vi "PDU Test Program.vi"() -> ()   [LabVIEW 2022 SP3, in "Power Distribution.lvclass"]
uses:
  Power Distribution.lvclass
  Orion PDU/Orion PDU.lvclass
  Power Distribution.lvclass/Power Distribution.ctl
panel:
  in  "Set":bool
  in  "Refresh Button":bool
  in  "stop":bool
  in  "States":bool[](array[boolean])
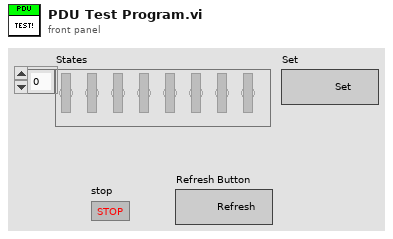
[diagram p1: front panel]
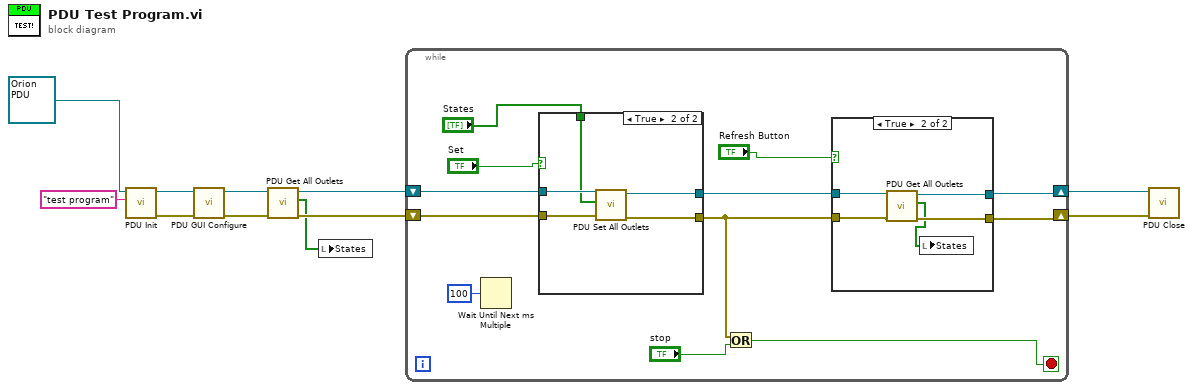
[diagram p0: block diagram]
diagram:
  n1 = call-dynamic "PDU Init.vi"("Name"="test program", "Orion PDU in"=refnum<class "Orion PDU.lvclass"> refnum ("Orion PDU.lvclass")) -> ("error out"=w2:errorcluster, "Orion PDU out"=w4:refnum<class "Orion PDU.lvclass">)  [unwired: 8 in]
  n2 = call-dynamic "PDU GUI Configure.vi"("error in (no error)"=w2, "Orion PDU in"=w4) -> ("error out"=w1:errorcluster, "Orion PDU out"=w3:refnum<class "Orion PDU.lvclass">)  [unwired: 8 in]
  n3 = call-dynamic "PDU Get All Outlets.vi"("error in (no error)"=w1, "Orion PDU in"=w3) -> ("error out"=w9:errorcluster, "States"=w8:bool[], "Orion PDU out"=w10:refnum<class "Orion PDU.lvclass">)  [unwired: 7 in]
  n4 = local write "States"(w8) -> ()
  n5 = while {
    shift-right: [w13] -> w6
    shift-left: w10 -> [w23]
    shift-right: [w14] -> w7
    shift-left: w9 -> [w21]
    stop <- w20 stop-if-true
    n6 = Wait Until Next ms Multiple(millisecond multiple=u32 100) -> ()  [unwired: 1 out]
    n7 = case shown="True" "Set" {
      tunnel: w23 -> [w32 w37]
      tunnel: "States" -> [_ w36]
      tunnel: w21 -> [w31 w35]
      tunnel: [w32 w34] -> w16
      tunnel: [w31 w33] -> w15
      frame False {
      }
      frame True {
        n8 = call-dynamic "PDU Set All Outlets.vi"("error in (no error)"=w35, "State"=w36, "Orion PDU in"=w37) -> ("error out"=w33:errorcluster, "Orion PDU out"=w34:refnum<class "Orion PDU.lvclass">)  [unwired: 7 in]
      }
    }
    n9 = Or(x=w15, y="stop") -> (x .or. y?=w20:bool)
    n10 = case shown="True" "Refresh Button" {
      tunnel: w16 -> [w25 w30]
      tunnel: w15 -> [w24 w29]
      tunnel: [w24 w28] -> w14
      tunnel: [w25 w27] -> w13
      frame False {
      }
      frame True {
        n11 = call-dynamic "PDU Get All Outlets.vi"("error in (no error)"=w29, "Orion PDU in"=w30) -> ("error out"=w28:errorcluster, "States"=w26:bool[], "Orion PDU out"=w27:refnum<class "Orion PDU.lvclass">)  [unwired: 7 in]
        n12 = local write "States"(w26) -> ()
      }
    }
  }
  n13 = call-dynamic "PDU Close.vi"("error in (no error)"=w7, "Orion PDU in"=w6) -> ()  [unwired: 8 in, 2 out]
